vi "Read Serial Number.vi"(0 "Session Handle in":T1, 11 "error in (no error)":errorcluster) -> (4 "Session Handle out":T1, 6 "Serial Number":string, 15 "error out":errorcluster)   [LabVIEW 2015, in "PAS.lvclass"]
uses:
  PAS.lvclass
  Typedefs/Session Handle.ctl
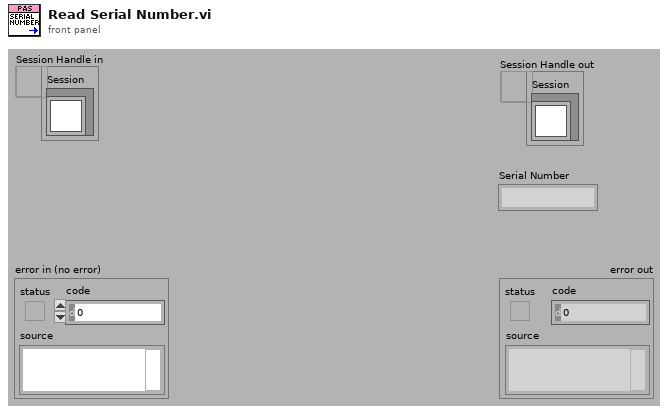
[diagram p1: front panel]
types:
  T1 = typedef "PAS.lvclass/Session Handle.ctl" = refnum<data-value>
  T2 = typedef "XNET Frame CAN.ctl" = cluster{"timestamp":timestamp, "payload":u8[], "identifier":u32, "type":T3, "extended?":bool, "echo?":bool}
  T3 = typedef "XNET Frame Type CAN.ctl" = u8
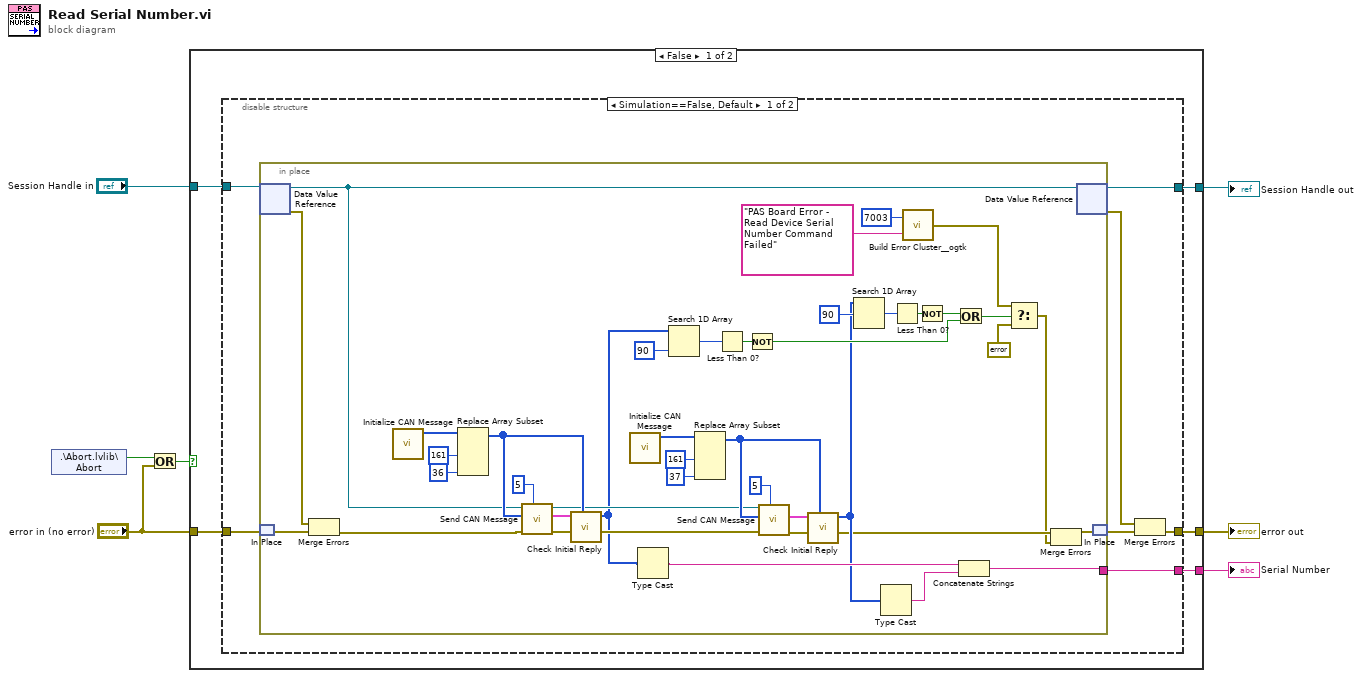
[diagram p0: block diagram]
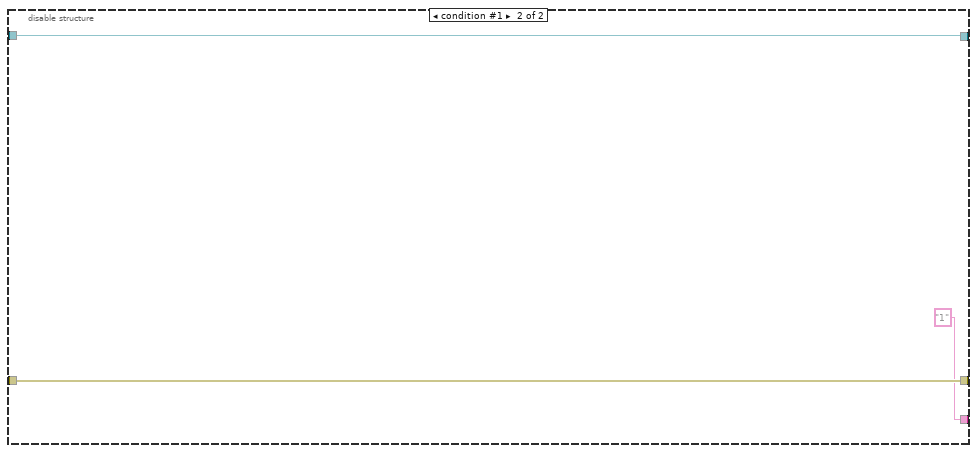
[diagram p2: hidden frame]
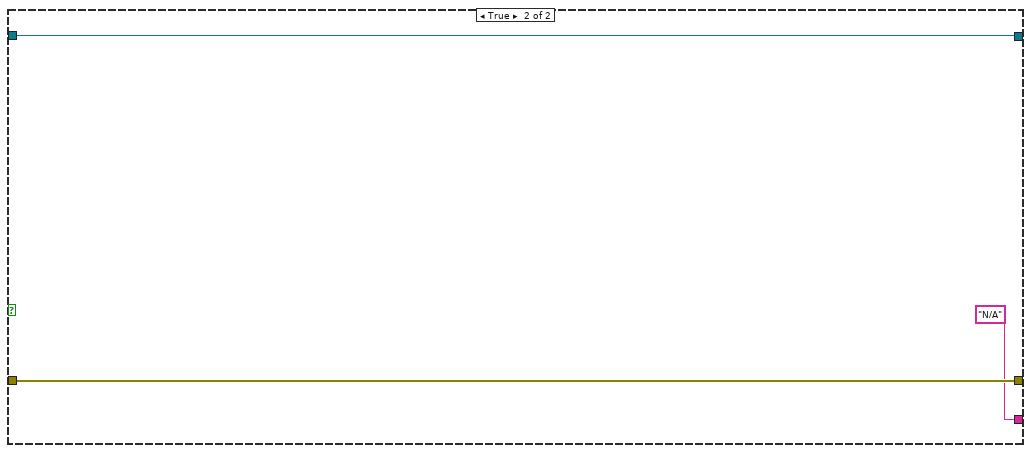
[diagram p3: hidden frame]
diagram:
  n1 = shared-variable ".\\Abort.lvlib\\Abort"() -> (w4:bool)  [unwired: 1 in, 1 out]
  n2 = Or(x=w4, y="error in (no error)") -> (x .or. y?=w2:bool)
  n3 = case shown="False" w2 {
    tunnel: [w12 w64] -> w6
    tunnel: [w11 w63] -> w5
    tunnel: "Session Handle in" -> [w10 w64]
    tunnel: "error in (no error)" -> [w9 w63]
    tunnel: [w8 "N/A"] -> w1
    frame False {
      n4 = disable-structure shown="Simulation==False, Default" {
        disable-tunnel: [w19 w61] -> w12
        disable-tunnel: [w16 w60] -> w11
        disable-tunnel: w10 -> [w15 w61]
        disable-tunnel: w9 -> [w14 w60]
        disable-tunnel: [w13 "1"] -> w8
        frame condition #0 (active) {
          n5 = in-place {
            in-place-border: [w33] -> w13
            n6 = in-place-dvr #1(w15) -> (w34:refnum<class "PAS.lvclass">, w57:errorcluster)
            n7 = in-place-match #2(w14) -> (w56:errorcluster)
            n8 = Merge Errors(w57, w56) -> (w35:errorcluster)
            n9 = call "Initialize CAN Message.vi"() -> ("Initial Payload"=w55:u8[])  [unwired: 11 in]
            n10 = Replace Array Subset(array=w55, new element #1=u8 161 ("new element/subarray"), new element #2=u8 36 ("new element/subarray")) -> (w50:u8[])  [unwired: 2 in]
            n11 = call "Send CAN Message.vi"("Number of Retries"=5, "error in (no error)"=w35, "payload"=w50, "Gas In"=w34) -> ("error out"=w42:errorcluster, "Reply"=w51:T2[], "Gas Out"=w43:refnum<class "PAS.lvclass">)  [unwired: 5 in]
            n12 = call "Check Initial Reply.vi"("Write Message"=w50, "Reply"=w51) -> ("Data Packet"=w25:u8[])  [unwired: 7 in, 2 out]
            n13 = call "Initialize CAN Message.vi"() -> ("Initial Payload"=w44:u8[])  [unwired: 11 in]
            n14 = Type Cast(x=w25) -> (*(type *) &x=w24:string)  [unwired: 1 in]
            n15 = Search 1D Array(1D array=w25, element=u8 90 ("new element/subarray")) -> (index of element=w40:i32)  [unwired: 1 in]
            n16 = Replace Array Subset(array=w44, new element #1=u8 161 ("new element/subarray"), new element #2=u8 37 ("new element/subarray")) -> (w49:u8[])  [unwired: 2 in]
            n17 = Less Than 0?(x=w40) -> (x < 0?=w36:bool)
            n18 = Not(x=w36) -> (.not. x?=w27:bool)
            n19 = call "Send CAN Message.vi"("Number of Retries"=5, "error in (no error)"=w42, "payload"=w49, "Gas In"=w43) -> ("error out"=w21:errorcluster, "Reply"=w48:T2[])  [unwired: 5 in, 1 out]
            n20 = call "Check Initial Reply.vi"("Write Message"=w49, "Reply"=w48) -> ("Data Packet"=w23:u8[])  [unwired: 7 in, 2 out]
            n21 = Search 1D Array(1D array=w23, element=u8 90 ("new element/subarray")) -> (index of element=w39:i32)  [unwired: 1 in]
            n22 = Type Cast(x=w23) -> (*(type *) &x=w22:string)  [unwired: 1 in]
            n23 = Less Than 0?(x=w39) -> (x < 0?=w37:bool)
            n24 = call <userlib>:"Build Error Cluster__ogtk.vi"("String to Prepend to source (\"\")"="PAS Board Error - Read Device Serial Number Command Failed" ("string"), "code"=7003) -> ("error out"=w29:errorcluster)
            n25 = Not(x=w37) -> (.not. x?=w26:bool)
            n26 = Or(x=w26, y=w27) -> (x .or. y?=w30:bool)
            n27 = Concatenate Strings(w24, w22) -> (w33:string)
            n28 = Select(t=w29, s=w30, f=errorcluster {"status"=FALSE, "code"=0, "source"=""}) -> (s? t:f=w20:errorcluster)
            n29 = Merge Errors(w21, w20) -> (w58:errorcluster)
            n30 = in-place-dvr #1(w34) -> (w19:T1, w17:errorcluster)
            n31 = in-place-match #2(w58) -> (w18:errorcluster)
          }
          n32 = Merge Errors(w17, w18) -> (w16:errorcluster)
        }
        frame condition #1 {
        }
      }
    }
    frame True {
    }
  }
  "Session Handle out" <- w6
  "error out" <- w5
  "Serial Number" <- w1
